vi "AI redefine.vi"(6 "conninfo":T4={"host"="localhost", "port"="5432", "client_encoding"="WIN1251", "dbname"="data", "user"="postgres", "password"=""}, 7 "KFM":string[](array[string]), 8 "error in (no error)":errorcluster, 9 "AIParamTable":string="fa_3", 10 "AIParameters":string[](array[string]), 11 "AI in":T1) -> (0 "error":errorcluster, 3 "AI out":T1)   [LabVIEW 2019, in "Inputs.lvlib"]
uses:
  Inputs.lvlib
  Ctl/AI.ctl
  Ctl/AI short.ctl
  Ctl/Parameter State.ctl
  Database/ctl/Coninfo.ctl
  Ctl/AIParamColumns.ctl
  Database/PostgreSQL2LabVIEW/libpqUtility/src/PQconnect.vi
  Database/PostgreSQL2LabVIEW/libpqUtility/src/PQclose.vi
  Database/select_initial_all.vi
  Database/PostgreSQL2LabVIEW/libpqlv/src/PQfinish.vi
  Database/PostgreSQL2LabVIEW/libpqlv/src/PQconnectdb.vi
  Database/PostgreSQL2LabVIEW/libpqlv/src/PQerrorMessage.vi
  Database/PostgreSQL2LabVIEW/libpqlv/src/PQstatus.vi
  <vilib>/dlg_ctls.llb/Space Constant.vi
  Database/PostgreSQL2LabVIEW/libpqUtility/src/PQgetTable.vi
  Database/Progress.vi
  Database/PostgreSQL.lvlib
panel:
  # "Analog parameters"
  # "Description of analog parameters"
  # "Analog parameters"
  # "Description of analog parameters"
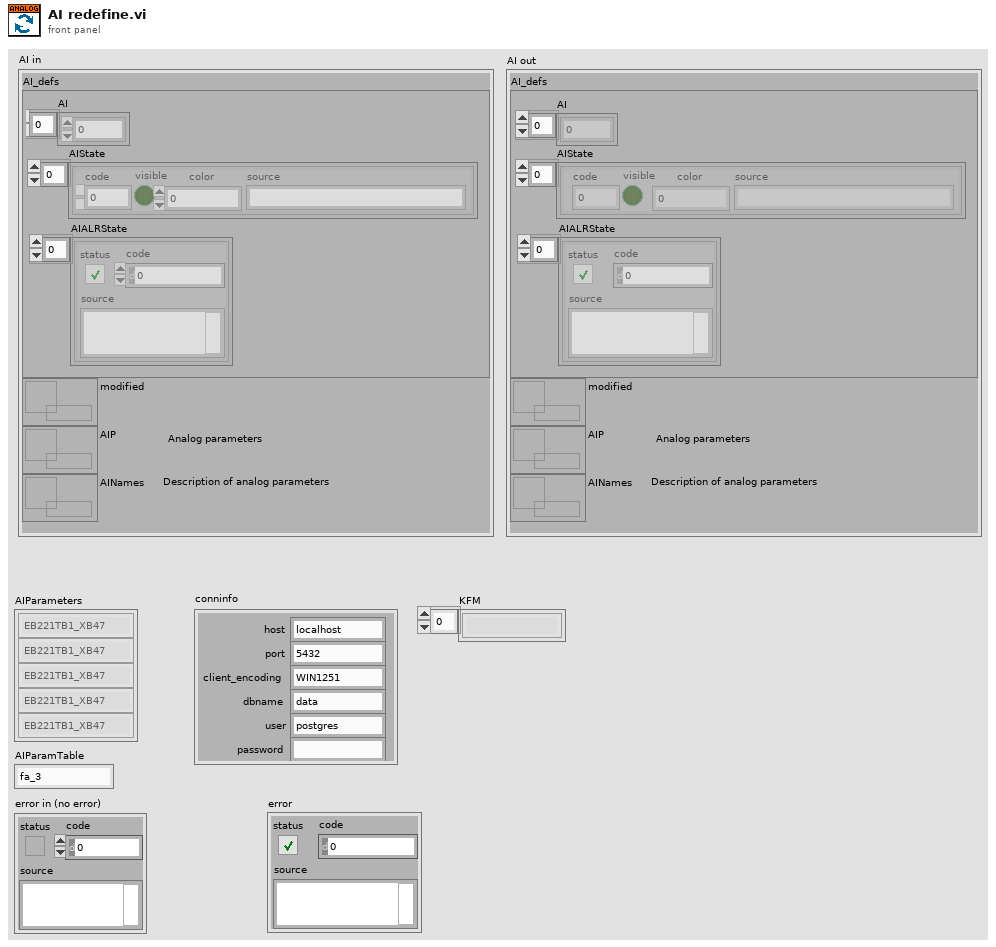
[diagram p1: front panel]
types:
  T1 = typedef "Inputs.lvlib/AI.ctl" = cluster{"AI_defs":T2, "modified":refnum<data-value>, "AIP":refnum<data-value>, "AINames":refnum<data-value>}
  T2 = typedef "Inputs.lvlib/AI short.ctl" = cluster{"AI":dbl[], "AIState":T3[], "AIALRState":errorcluster[]}
  T3 = typedef "Inputs.lvlib/Parameter State.ctl" = cluster{"code":i32, "visible":bool, "color":u32, "source":string}
  T4 = typedef "PostgreSQL.lvlib/Coninfo.ctl" = cluster{"host":string, "port":string, "client_encoding":string, "dbname":string, "user":string, "password":string}
  T5 = typedef "Inputs.lvlib/AIParamColumns.ctl" = enum16{"instrument_gain", "instrument_offset", "time_const", "instrument_min_offset", "instrument_range_min", "process_range_min", "process_low_acd", "process_low_alr", "process_high_alr", "process_high_acd", "process_range_max", "instrument_range_max", "instrument_max_offset", "d", "input_register_min", "input_register_max", "input_pv_min", "input_pv_max", "module_fcode_full", "control_channel_num", "ip_adress", "fcode", "fcodef", "fcode_full", "fname", "process_units"}
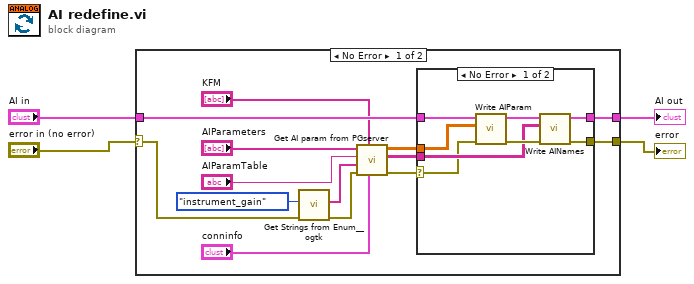
[diagram p0: block diagram]
diagram:
  n1 = case shown="No Error" "error in (no error)" {
    selector: "error in (no error)" -> [w6 w30]
    tunnel: [w13 w30] -> w4
    tunnel: "AI in" -> [w11 w29]
    tunnel: [w10 w29] -> w3
    frame No Error {
      n2 = call <userlib>:"Get Strings from Enum__ogtk.vi"("error in (no error)"=w6, "Enum"=AIParamColumns."instrument_gain" ("AIParamColumns")) -> ("error out"=w5:errorcluster, "Enum Strings"=w7:string[])  [unwired: 6 in, 2 out]
      n3 = call "Get AI param from PGserver.vi"("conninfo"="conninfo", "KFM"="KFM", "error in (no error)"=w5, "AIParamColumns"=w7, "AIParamTable"="AIParamTable", "AIParameters"="AIParameters") -> ("error out"=w15:errorcluster, "Names table"=w16:string[][], "Parameters table"=w17:dbl[][])  [unwired: 3 in]
      n4 = case shown="No Error" w15 {
        selector: w15 -> [w19 w27]
        tunnel: w17 -> [w21 _]
        tunnel: w16 -> [w20 _]
        tunnel: [w23 w27] -> w13
        tunnel: w11 -> [w26 w28]
        tunnel: [w22 w28] -> w10
        frame No Error {
          n5 = call "Write AIParam.vi"("error in (no error)"=w19, "AIParam"=w21, "AI in"=w26) -> ("error out"=w24:errorcluster, "AI out"=w25:T1)  [unwired: 7 in]
          n6 = call "Write AINames.vi"("error in (no error)"=w24, "ALRNames"=w20, "AI in"=w25) -> ("error out"=w23:errorcluster, "AI out"=w22:T1)  [unwired: 7 in]
        }
        frame Error {
        }
      }
    }
    frame Error {
    }
  }
  "AI out" <- w3
  "error" <- w4
